vi "one element of zero (DBL).vi"(10 "Array in":dbl[](array[numeric])) -> (2 "equal [0]?":bool)   [LabVIEW 2018, in "NI_AALPro.lvlib"]
uses:
  <vilib>/Analysis/NI_AALPro.lvlib
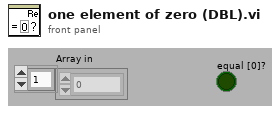
[diagram p1: front panel]
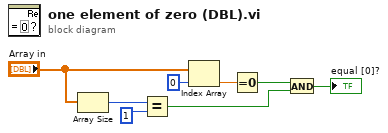
[diagram p0: block diagram]
diagram:
  n1 = Array Size(array="Array in") -> (size(s)=w7:i32)
  n2 = Equal?(x=w7, y=1) -> (x = y?=w2:bool)
  n3 = Index Array(array="Array in", index=0) -> (element=w4:dbl)
  n4 = Equal To 0?(x=w4) -> (x = 0?=w3:bool)
  n5 = And(x=w3, y=w2) -> (x .and. y?=→"equal [0]?":bool)
